vi "Append Control Image.vi"(0 "PDF Report IN":refnum<class "PDF Report Class.lvclass">, 1 "Scale (%)":sgl=100.0, 3 "Border":T3={"Show?"=FALSE, "Thickness (point)"=0.5, "Color"=0}, 5 "Ctrl reference":refnum<vi>, 11 "error in (no error)":errorcluster, 12 "Caption":string, 14 "Position and indentation":T1={"Alignment"=enum."Center", "X "=0.0, "Y"=0.0, "Indentation"=0.0}) -> (4 "PDF Report OUT":refnum<class "PDF Report Class.lvclass">, 15 "error out":errorcluster)   [LabVIEW 2019, in "Exaprom PDF.lvlib"]
doc: "Creates an image of the front panel object specified in <B>Ctrl reference</B> and appends it to a PDF report.\n\n<B>FRANÇAIS</B>\nCréation de l'image d'un objet du panneau avant spécifié par <B>Ctrl reference</B> et ajout au rapport PDF.\n\nVersion 1.0\nDeveloped by Jean-Marc Simard\nCopyright © 2010, Exaprom Inc.\nAll rights reserved.\nLicense: BSD\n\nWith iTextSharp 4.1.6 (http://itextsharp.sourceforge.net)\nunder Mozilla Public License Version 1.1\n(http://www.mozilla.org/MPL/MPL-1.1.html)"
uses:
  LV Class/PDF Report Class/PDF Report Class.lvclass
  Controls/Image Controls/Image border.ctl
  Controls/Image Controls/Image alignment and position.ctl
  Controls/Image Controls/Image aligment.ctl
  C:/work/niobrara_lv/labview pdf writer fixing/DLL/itextsharp.dll
  DLL/itextsharp.dll
  Exaprom PDF.lvlib
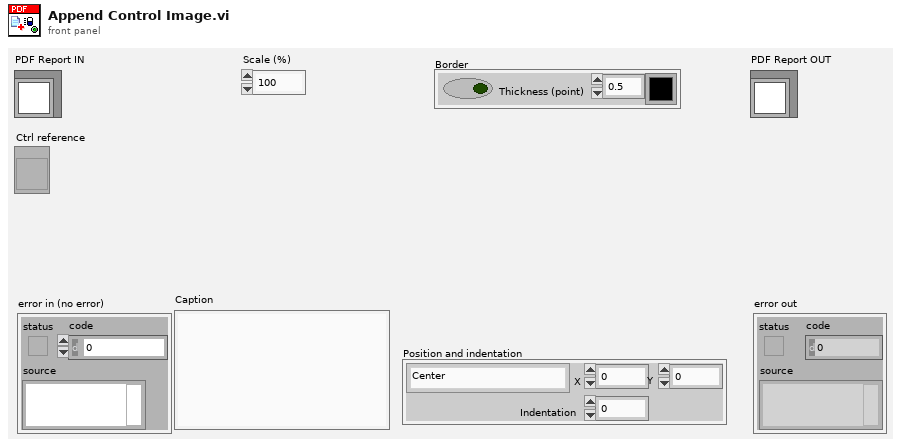
[diagram p1: front panel]
types:
  T1 = typedef "Exaprom PDF.lvlib/Image alignment and position.ctl" = cluster{"Alignment":T2, "X ":sgl, "Y":sgl, "Indentation":sgl}
  T2 = typedef "Exaprom PDF.lvlib/Image aligment.ctl" = enum16{"Absolute (X,Y)", "Left", "Center", "Right", "Left (textwrap)", "Right (textwrap)"}
  T3 = typedef "Exaprom PDF.lvlib/Image border.ctl" = cluster{"Show?":bool, "Thickness (point)":sgl, "Color":u32}
  T4 = typedef "imagedata.ctl" = cluster{"image type":i32, "image depth":i32, "image":u8[], "mask":u8[], "colors":u32[], "Rectangle":cluster{"left":i16, "top":i16, "right":i16, "bottom":i16}}
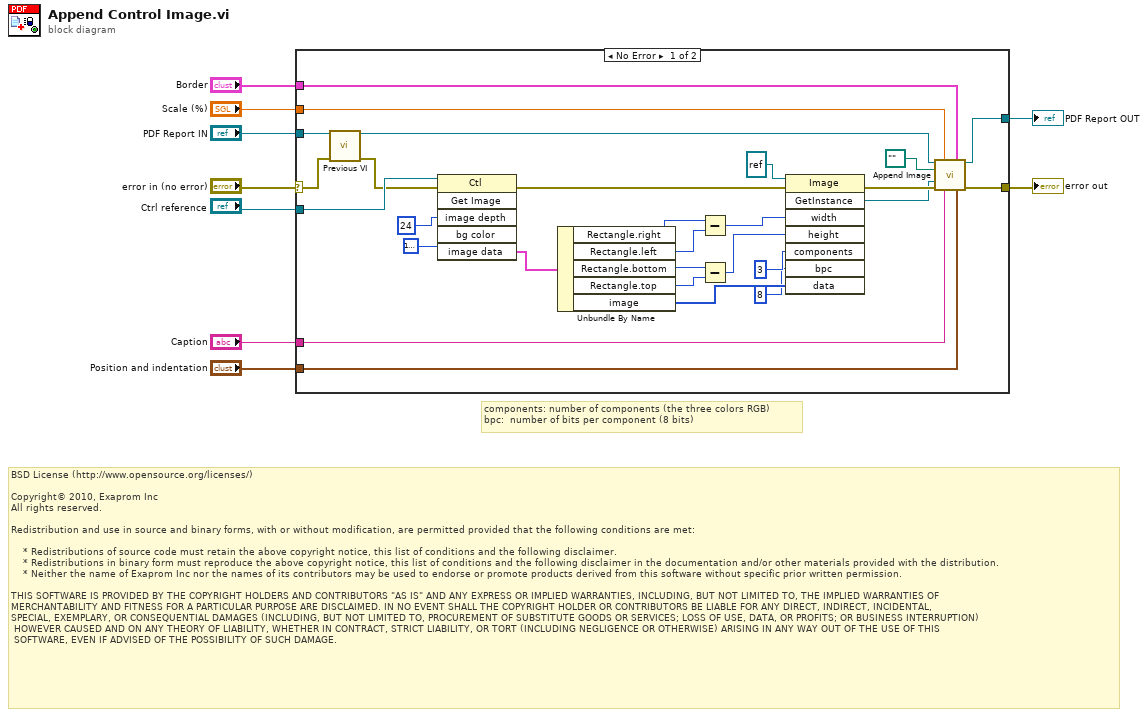
[diagram p0: block diagram]
diagram:
  # "components: number of components (the three colors RGB)\nbpc:  number of bits per component (8 bits)"
  # "BSD License (http://www.opensource.org/licenses/)\n\nCopyright© 2010, Exaprom Inc\nAll rights reserved.\n\nRedistribution and use in source and binary forms, with or without modification, are permitted provided that the following conditions are met:\n\n    * Redistributions of source code must retain the above copyright notice, this list of conditions and the following disclaimer.\n    * Redistributions in binary form must reproduce the above copyright notice, this list of conditions and the following disclaimer in the documentation and/or other materials provided with the distribution.\n    * Neither the name of Exaprom Inc nor the names of its contributors may be used to endorse or promote products derived from this software without specific prior written permission.\n\nTHIS SOFTWARE IS PROVIDED BY THE COPYRIGHT HOLDERS AND CONTRIBUTORS \"AS IS\" AND ANY EXPRESS OR IMPLIED WARRANTIES, INCLUDING, BUT NOT LIMITED TO, THE IMPLIED WARRANTIES OF \nMERCHANTABILITY AND FITNESS FOR A PARTICULAR PURPOSE ARE DISCLAIMED. IN NO EVENT SHALL THE COPYRIGHT HOLDER OR CONTRIBUTORS BE LIABLE FOR ANY DIRECT, INDIRECT, INCIDENTAL,\nSPECIAL, EXEMPLARY, OR CONSEQUENTIAL DAMAGES (INCLUDING, BUT NOT LIMITED TO, PROCUREMENT OF SUBSTITUTE GOODS OR SERVICES; LOSS OF USE, DATA, OR PROFITS; OR BUSINESS INTERRUPTION)\n HOWEVER CAUSED AND ON ANY THEORY OF LIABILITY, WHETHER IN CONTRACT, STRICT LIABILITY, OR TORT (INCLUDING NEGLIGENCE OR OTHERWISE) ARISING IN ANY WAY OUT OF THE USE OF THIS\n SOFTWARE, EVEN IF ADVISED OF THE POSSIBILITY OF SUCH DAMAGE."
  n1 = case shown="No Error" "error in (no error)" {
    selector: "error in (no error)" -> [w11 w39]
    tunnel: [w18 w39] -> w7
    tunnel: "Ctrl reference" -> [w36 _]
    tunnel: [w32 w38] -> w6
    tunnel: "PDF Report IN" -> [w33 w38]
    tunnel: "Caption" -> [w17 _]
    tunnel: "Position and indentation" -> [w16 _]
    tunnel: "Border" -> [w15 _]
    tunnel: "Scale (%)" -> [w14 _]
    frame No Error {
      n2 = call "Previous VI.vi"("PDF Report IN"=w33, "error in (no error)"=w11) -> ("PDF Report OUT"=w12:refnum<class "PDF Report Class.lvclass">, "error out"=w10:errorcluster)  [unwired: 12 out]
      n3 = invoke class="Ctl" method="Get Image"(reference=w36, error in=w10, "image depth"=24 ("Image Depth"), "bg color"=u32 16777225) -> (error out=w37:errorcluster, "image data"=w31:T4)  [unwired: 2 in, 4 out]
      n4 = Unbundle By Name(w31) -> ("Rectangle.right"=w27:i16, "Rectangle.left"=w26:i16, "Rectangle.bottom"=w24:i16, "Rectangle.top"=w23:i16, "image"=w20:u8[])
      n5 = Subtract(x=w27, y=w26) -> (x-y=w25:i16)
      n6 = Subtract(x=w24, y=w23) -> (x-y=w22:i16)
      n7 = invoke class="Image" method="GetInstance"(reference=refnum<k24> refnum ("image"), error in=w37, "width"=w25, "height"=w22, "components"=3, "bpc"=8, "data"=w20) -> (error out=w34:errorcluster, "GetInstance"=w13:refnum<k24>)  [unwired: 1 in, 6 out]
      n8 = call "Append Image.vi"("PDF Report IN"=w12, "Scale (%)"=w14, "Border"=w15, "Image path"=path "" ("path"), "Image Ref iTexSharp"=w13, "error in (no error)"=w34, "Caption"=w17, "Position and indentation"=w16) -> ("PDF Report OUT"=w32:refnum<class "PDF Report Class.lvclass">, "error out"=w18:errorcluster)  [unwired: 6 out]
    }
    frame Error {
    }
  }
  "error out" <- w7
  "PDF Report OUT" <- w6
